vi "Set Phase.vi"(8 "error in (no error)":errorcluster, 9 "phase":dbl[unit], 10 "Channel (0: Channel 1)":T1 items=["Channel 1", "Channel 2"], 11 "VISA resource name":refnum<visa-resource-name>) -> (0 "error out":errorcluster, 3 "VISA resource name out":refnum<visa-resource-name>)   [LabVIEW 2012, in "Tektronix AFG 3000 Series.lvlib"]
doc: "Sets the phase of a Tektronix AFG 3000 series function generator. May not be used with the waveforms DC, Noise, or Pulse."
uses:
  Tektronix AFG 3000 Series.lvlib
  controls.llb/Channel.ctl
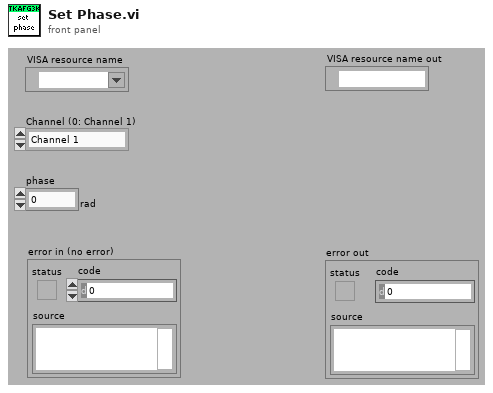
[diagram p1: front panel]
types:
  T1 = typedef "Channel.ctl" = u16
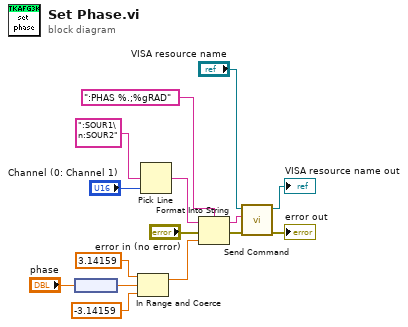
[diagram p0: block diagram]
diagram:
  n1 = node("phase") -> (w2:dbl)
  n2 = In Range and Coerce(upper limit=3.14159, x=w2, lower limit=-3.14159) -> (coerced(x)=w5:dbl)  [unwired: 1 out]
  n3 = Pick Line(multi-line string=":SOUR1\n:SOUR2", line index="Channel (0: Channel 1)") -> (output string=w12:string)  [unwired: 1 out]
  n4 = Format Into String(format string=":PHAS %.;%gRAD", initial string=w12, error in="error in (no error)", w5) -> (resulting string=w1:string, error out=w9:errorcluster)
  n5 = call "Send Command.vi"("error in (no error)"=w9, "write buffer"=w1, "VISA resource name"="VISA resource name") -> ("error out"=→"error out":errorcluster, "VISA resource name out"=→"VISA resource name out":refnum<visa-resource-name>)  [unwired: 7 out]
